vi "Image Manager for Grab Acquisition.vi"(7 "Mode":T4, 8 "error in (no error)":errorcluster, 9 "Init Settings":T3={"Number of Processing Images"=1, "Image Border Size"=0} {"Number of Processing Images" min=1 max=1000}, 10 "Image Settings In":cluster{"Image":T1, "Buffer Number":u32}, 11 "Session In":T2) -> (0 "error out":errorcluster, 1 "No Available Image":bool, 2 "Image Settings Out":cluster{"Image":T1, "Buffer Number":u32}, 3 "Session Out":T2)   [LabVIEW 2018]
uses:
  <vilib>/vision/Image Controls.llb/IMAQ Image.ctl
  Grab Manager Mode.ctl
  <vilib>/userDefined/High Color/IMAQdx.ctl
panel:
  in  "Invalid Image":errorcluster={"status"=TRUE, "code"=-2, "source"="The image passed in is not valid to Unlockl"}
  in  "Invalid Session":errorcluster={"status"=TRUE, "code"=-1, "source"="The images for this session are not available anymore."}
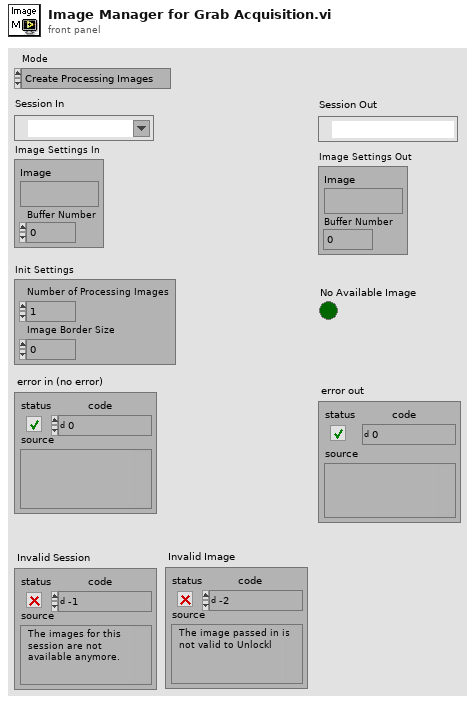
[diagram p1: front panel]
types:
  T1 = typedef "IMAQ Image.ctl" = refnum<image>
  T2 = typedef "IMAQdx.ctl" = refnum<k21>
  T3 = cluster{"Number of Processing Images":u32, "Image Border Size":u32}
  T4 = typedef "Grab Manager Mode.ctl" = enum16{"Create Processing Images", "Lock", "Add Acquired Image", "Get Acquired Image", "Unlock", "Dispose Processing Images"}
  T5 = cluster{cluster{"Image":T1, "Buffer Number":u32}[]}
  T6 = cluster{cluster{"Image":T1, "Buffer Number":u32}[]}[]
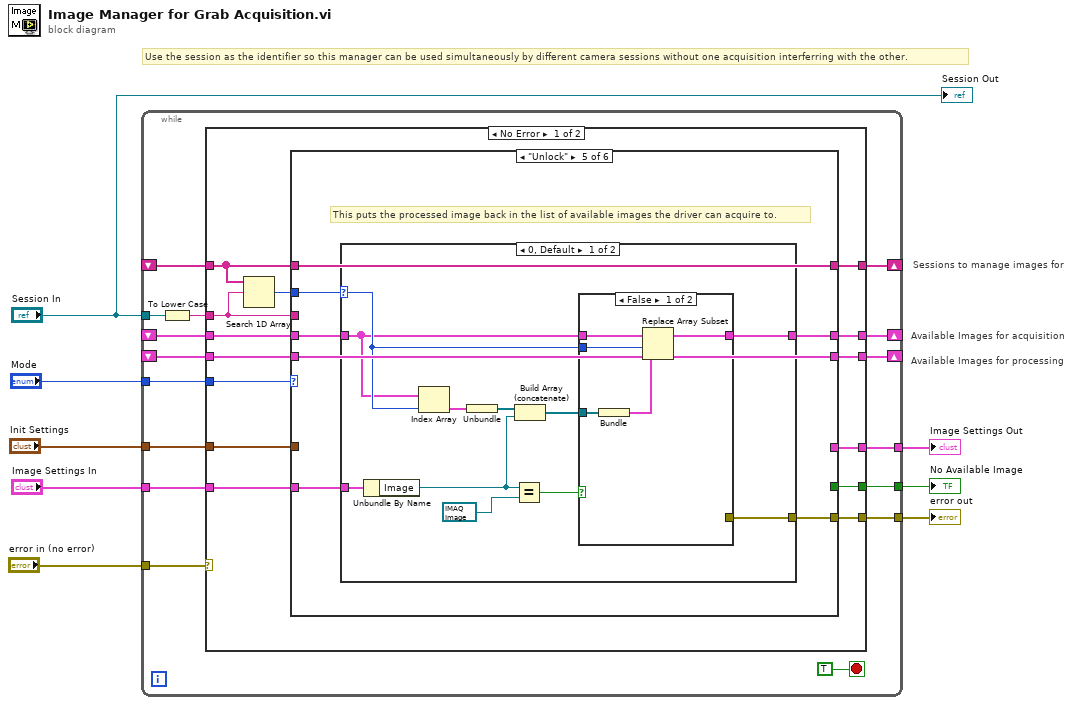
[diagram p0: block diagram]
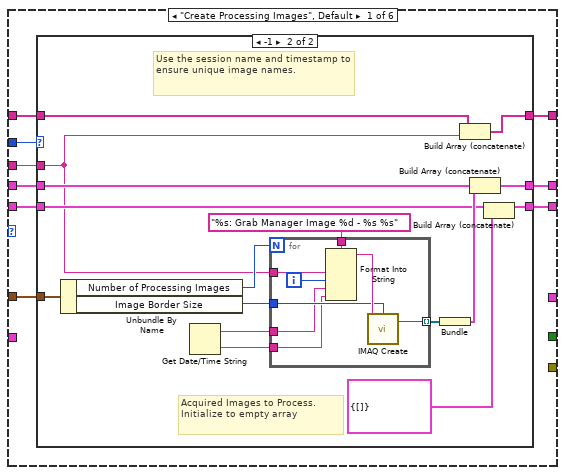
[diagram p2: hidden frame]
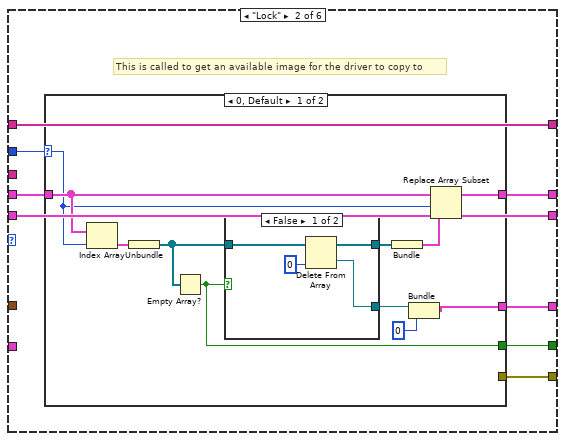
[diagram p4: hidden frame]
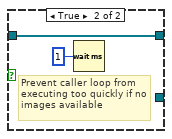
[diagram p5: hidden frame]
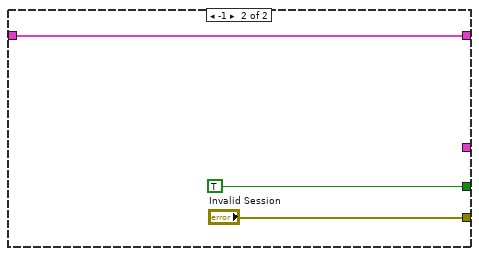
[diagram p6: hidden frame]
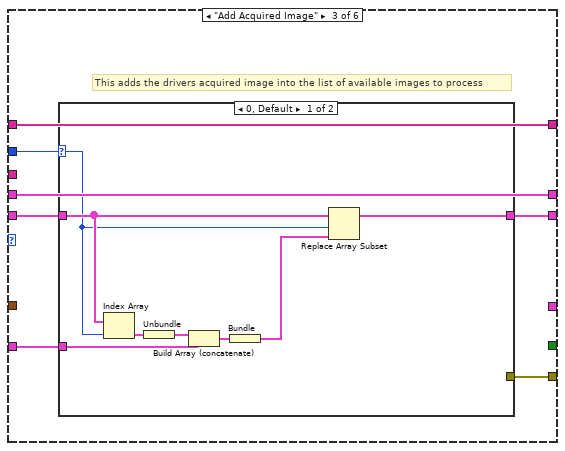
[diagram p7: hidden frame]
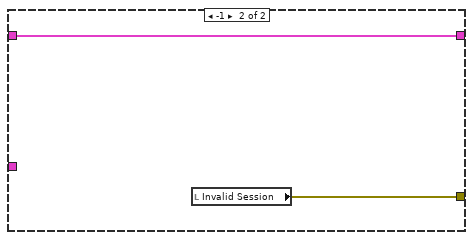
[diagram p8: hidden frame]
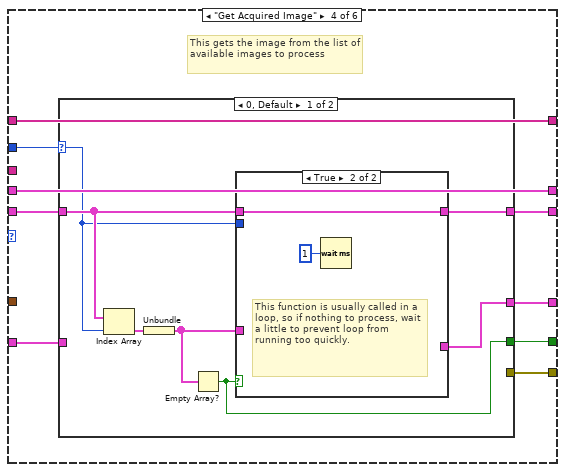
[diagram p9: hidden frame]
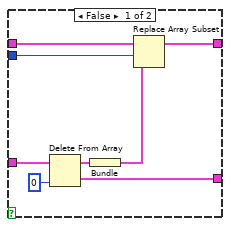
[diagram p10: hidden frame]
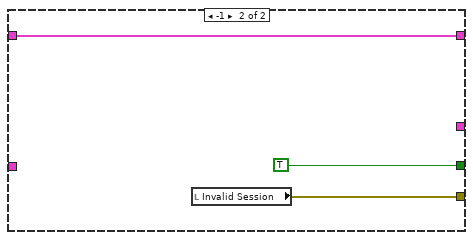
[diagram p11: hidden frame]
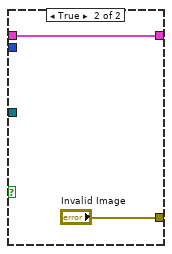
[diagram p12: hidden frame]
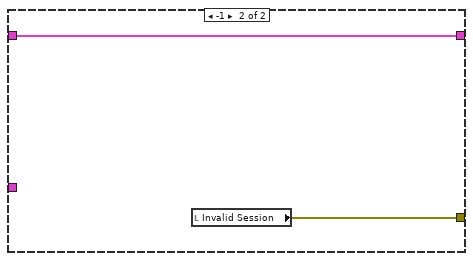
[diagram p13: hidden frame]
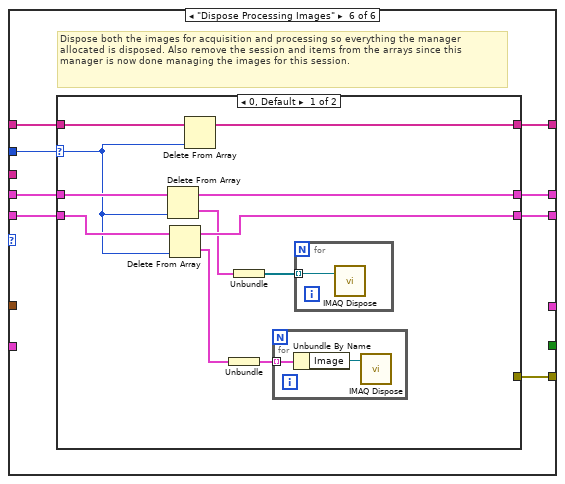
[diagram p14: hidden frame]
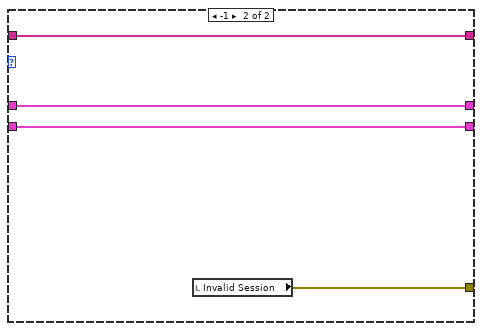
[diagram p15: hidden frame]
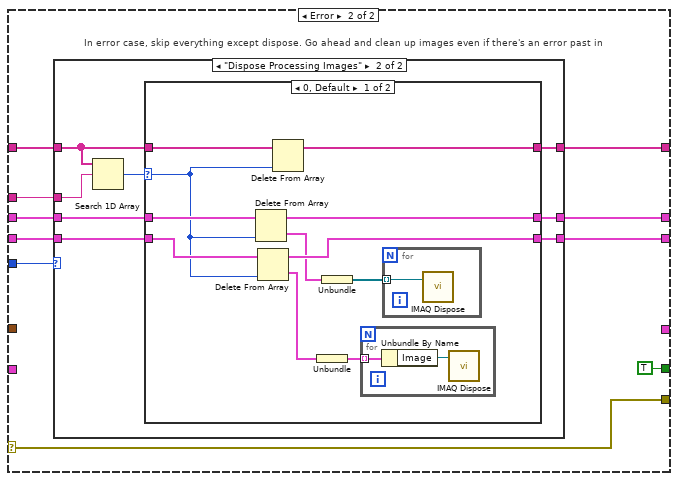
[diagram p16: hidden frame]
diagram:
  # "Use the session as the identifier so this manager can be used simultaneously by different camera sessions without one acquisition interferring with the other."
  # "Available Images for processing"
  # "Available Images for acquisition"
  # "Sessions to manage images for"
  n1 = while {
    tunnel: "Mode" -> [w24]
    tunnel: [w23] -> w7
    tunnel: "Session In" -> [w22]
    tunnel: "error in (no error)" -> [w20]
    tunnel: "Init Settings" -> [w19]
    shift-right: [w18] -> _
    shift-left: _ -> [w17]
    shift-right: [w16] -> _
    shift-left: _ -> [w15]
    tunnel: [w14] -> w3
    shift-right: [w13] -> _
    shift-left: _ -> [w12]
    tunnel: [w11] -> w1
    tunnel: "Image Settings In" -> [w10]
    stop <- TRUE stop-if-true
    n2 = To Lower Case(string=w22) -> (all lower case string=w9:string)
    n3 = case shown="No Error" w20 {
      selector: w20 -> [_ w211]
      tunnel: w24 -> [w38 w203]
      tunnel: [w37 _] -> w11
      tunnel: [w28 w211] -> w14
      tunnel: [w36 TRUE ("empty?")] -> w23
      tunnel: w9 -> [w34 w209]
      tunnel: w19 -> [w35 _]
      tunnel: [w33 w206] -> w18
      tunnel: w17 -> [w32 w210]
      tunnel: [w30 w205] -> w16
      tunnel: w15 -> [w29 w208]
      tunnel: [w27 w204] -> w13
      tunnel: w12 -> [w26 w207]
      tunnel: w10 -> [w25 _]
      frame No Error {
        n4 = Search 1D Array(1D array=w32, element=w34) -> (index of element=w31:i32)  [unwired: 1 in]
        n5 = case shown="\"Unlock\"" w38 {
          tunnel: [_ w75 _ w121 _ _] -> w37
          tunnel: [_ w82 _ w120 _ _] -> w36
          tunnel: w34 -> [w46 _ _ _ _ _]
          tunnel: w35 -> [w47 _ _ _ _ _]
          tunnel: [w45 w80 w108 w127 w154 w179] -> w33
          tunnel: w32 -> [w44 w80 w108 w127 w154 w180]
          tunnel: w31 -> [w43 w81 w109 w128 w155 w183]
          tunnel: [w42 w78 w107 w126 w150 w178] -> w30
          tunnel: w29 -> [w41 w79 w107 w126 w151 w182]
          tunnel: [_ w77 w104 w123 w153 w176] -> w28
          tunnel: [w40 w76 w105 w124 w149 w177] -> w27
          tunnel: w26 -> [w39 w76 w106 w125 w149 w181]
          tunnel: w25 -> [_ _ w103 w122 w152 _]
          frame "Create Processing Images", Default {
            n6 = case shown="-1" w43 {
              tunnel: w47 -> [_ w66]
              tunnel: w46 -> [_ w53]
              tunnel: [w50 w65] -> w45
              tunnel: w44 -> [w50 w64]
              tunnel: [w49 w59] -> w42
              tunnel: w41 -> [w49 w58]
              tunnel: [w48 w56] -> w40
              tunnel: w39 -> [w48 w55]
              frame 0, Default {
                # "This session has already been initialized. Keep the same images"
              }
              frame -1 {
                # "Acquired Images to Process. Initialize to empty array"
                # "Use the session name and timestamp to ensure unique image names."
                n7 = Unbundle By Name(w66) -> ("Number of Processing Images"=w63:u32, "Image Border Size"=w62:u32)
                n8 = Get Date/Time String() -> (date string=w52:string, time string=w51:string)  [unwired: 3 in]
                n9 = for {
                  N: w63 -> [_]
                  tunnel: [w74] -> w61 mode=indexing
                  tunnel: w53 -> [w71]
                  tunnel: w62 -> [w70]
                  tunnel: "%s: Grab Manager Image %d - %s %s" ("Image Name") -> [w69]
                  tunnel: w52 -> [w68]
                  tunnel: w51 -> [w67]
                  i -> [w73]
                  n10 = Format Into String(format string=w69, w71, w73, w68, w67) -> (resulting string=w72:string)  [unwired: 2 in, 1 out]
                  n11 = call "IMAQ Create"("Border Size"=w70, "Image Name"=w72) -> ("New Image"=w74:T1)  [unwired: 2 in, 2 out]
                }
                n12 = Bundle(w61) -> (w60:cluster{T1[]})  [unwired: 1 in]
                n13 = Build Array (concatenate)(w64, w53) -> (w65:string[])
                n14 = Build Array (concatenate)(w58, w60) -> (w59:cluster{T1[]}[])
                n15 = Build Array (concatenate)(w55, T5 {[]}) -> (w56:T6)
              }
            }
          }
          frame "Lock" {
            # "This is called to get an available image for the driver to copy to"
            n16 = case shown="0, Default" w81 {
              selector: w81 -> [w87 _]
              tunnel: [w93 TRUE ("empty?")] -> w82
              tunnel: w79 -> [w89 w102]
              tunnel: [w88 w102] -> w78
              tunnel: [_ "Invalid Session"] -> w77
              tunnel: [w83 _] -> w75
              frame 0, Default {
                n17 = Index Array(array=w89, index=w87) -> (element=w92:cluster{T1[]})
                n18 = Unbundle(w92) -> (w91:T1[])
                n19 = Empty Array?(array=w91) -> (empty?=w93:bool)
                n20 = case shown="False" w93 {
                  tunnel: [w96 w99] -> w90
                  tunnel: [w95 _] -> w85
                  tunnel: w91 -> [w94 w99]
                  frame False {
                    n21 = Delete From Array(array=w94, index=0) -> (deleted portion=w95:T1, array with subset deleted=w96:T1[])  [unwired: 1 in]
                  }
                  frame True {
                    # "Prevent caller loop from executing too quickly if no images available"
                    n22 = Wait (ms)(milliseconds to wait=u32 1) -> ()  [unwired: 1 out]
                  }
                }
                n23 = Bundle(w90) -> (w86:cluster{T1[]})  [unwired: 1 in]
                n24 = Bundle("New Image"=w85, u32 0) -> (w83:cluster{"New Image":T1, u32})  [unwired: 1 in]
                n25 = Replace Array Subset(array=w89, new element=w86, index=w87) -> (w88:cluster{T1[]}[])
              }
              frame -1 {
              }
            }
          }
          frame "Add Acquired Image" {
            # "This adds the drivers acquired image into the list of available images to process"
            n26 = case shown="0, Default" w109 {
              selector: w109 -> [w112 _]
              tunnel: w106 -> [w115 w119]
              tunnel: [w111 w119] -> w105
              tunnel: [_ w118] -> w104
              tunnel: w103 -> [w110 _]
              frame 0, Default {
                n27 = Index Array(array=w115, index=w112) -> (element=w117:T5)
                n28 = Unbundle(w117) -> (w116:cluster{"Image":T1, "Buffer Number":u32}[])
                n29 = Build Array (concatenate)(w116, w110) -> (w114:cluster{"Image":T1, "Buffer Number":u32}[])
                n30 = Bundle(w114) -> (w113:T5)  [unwired: 1 in]
                n31 = Replace Array Subset(array=w115, new element=w113, index=w112) -> (w111:T6)
              }
              frame -1 {
                n32 = local read "Invalid Session"() -> (w118:errorcluster)
              }
            }
          }
          frame "Get Acquired Image" {
            # "This gets the image from the list of available images to process"
            n33 = case shown="0, Default" w128 {
              selector: w128 -> [w133 _]
              tunnel: w125 -> [w134 w148]
              tunnel: [w132 w148] -> w124
              tunnel: [_ w147] -> w123
              tunnel: w122 -> [_ _]
              tunnel: [w130 _] -> w121
              tunnel: [w129 TRUE ("empty?")] -> w120
              frame 0, Default {
                n34 = Index Array(array=w134, index=w133) -> (element=w135:T5)
                n35 = Unbundle(w135) -> (w131:cluster{"Image":T1, "Buffer Number":u32}[])
                n36 = Empty Array?(array=w131) -> (empty?=w129:bool)
                n37 = case shown="True" w129 {
                  tunnel: w134 -> [w143 w145]
                  tunnel: w133 -> [w142 _]
                  tunnel: [w141 w145] -> w132
                  tunnel: w131 -> [w139 _]
                  tunnel: [w136 _] -> w130
                  frame False {
                    n38 = Delete From Array(array=w139, index=0) -> (deleted portion=w136:cluster{"Image":T1, "Buffer Number":u32}, array with subset deleted=w138:cluster{"Image":T1, "Buffer Number":u32}[])  [unwired: 1 in]
                    n39 = Bundle(w138) -> (w137:T5)  [unwired: 1 in]
                    n40 = Replace Array Subset(array=w143, new element=w137, index=w142) -> (w141:T6)
                  }
                  frame True {
                    # "This function is usually called in a loop, so if nothing to process, wait a little to prevent loop from running too quickly."
                    n41 = Wait (ms)(milliseconds to wait=u32 1) -> ()  [unwired: 1 out]
                  }
                }
              }
              frame -1 {
                n42 = local read "Invalid Session"() -> (w147:errorcluster)
              }
            }
          }
          frame "Unlock" {
            # "This puts the processed image back in the list of available images the driver can acquire to."
            n43 = case shown="0, Default" w155 {
              selector: w155 -> [w165 _]
              tunnel: [w156 w175] -> w153
              tunnel: w152 -> [w166 _]
              tunnel: w151 -> [w161 w174]
              tunnel: [w160 w174] -> w150
              frame 0, Default {
                n44 = Unbundle By Name(w166) -> ("Image"=w159:T1)
                n45 = Index Array(array=w161, index=w165) -> (element=w164:cluster{T1[]})
                n46 = Unbundle(w164) -> (w163:T1[])
                n47 = Equal?(x=w159, y=T1 refnum) -> (x = y?=w157:bool)
                n48 = Build Array (concatenate)(w163, w159) -> (w162:T1[])
                n49 = case shown="False" w157 {
                  tunnel: w165 -> [w171 _]
                  tunnel: w162 -> [w169 _]
                  tunnel: w161 -> [w168 w173]
                  tunnel: [w167 w173] -> w160
                  tunnel: [_ "Invalid Image"] -> w156
                  frame False {
                    n50 = Bundle(w169) -> (w170:cluster{T1[]})  [unwired: 1 in]
                    n51 = Replace Array Subset(array=w168, new element=w170, index=w171) -> (w167:cluster{T1[]}[])
                  }
                  frame True {
                  }
                }
              }
              frame -1 {
                n52 = local read "Invalid Session"() -> (w175:errorcluster)
              }
            }
          }
          frame "Dispose Processing Images" {
            # "Dispose both the images for acquisition and processing so everything the manager allocated is disposed. Also remove the session and items from the arrays since this manager is now done managing the images for this session."
            n53 = case shown="0, Default" w183 {
              selector: w183 -> [w188 _]
              tunnel: w182 -> [w191 w199]
              tunnel: w181 -> [w189 w198]
              tunnel: w180 -> [w193 w200]
              tunnel: [w192 w200] -> w179
              tunnel: [w190 w199] -> w178
              tunnel: [w187 w198] -> w177
              tunnel: [_ w201] -> w176
              frame 0, Default {
                n54 = Delete From Array(array=w191, index=w188) -> (deleted portion=w186:cluster{T1[]}, array with subset deleted=w190:cluster{T1[]}[])  [unwired: 1 in]
                n55 = Delete From Array(array=w189, index=w188) -> (deleted portion=w185:T5, array with subset deleted=w187:T6)  [unwired: 1 in]
                n56 = Delete From Array(array=w193, index=w188) -> (array with subset deleted=w192:string[])  [unwired: 1 in, 1 out]
                n57 = Unbundle(w185) -> (w184:cluster{"Image":T1, "Buffer Number":u32}[])
                n58 = Unbundle(w186) -> (w194:T1[])
                n59 = for {
                  tunnel: w184 -> [w196] mode=indexing
                  n60 = Unbundle By Name(w196) -> ("Image"=w195:T1)
                  n61 = call "IMAQ Dispose"("Image"=w195) -> ()  [unwired: 5 in, 1 out]
                }
                n62 = for {
                  tunnel: w194 -> [w197] mode=indexing
                  n63 = call "IMAQ Dispose"("Image"=w197) -> ()  [unwired: 5 in, 1 out]
                }
              }
              frame -1 {
                n64 = local read "Invalid Session"() -> (w201:errorcluster)
              }
            }
          }
        }
      }
      frame Error {
        # "In error case, skip everything except dispose. Go ahead and clean up images even if there's an error past in"
        n65 = case shown="\"Dispose Processing Images\"" w203 {
          tunnel: w210 -> [w214 w222]
          tunnel: w209 -> [_ w221]
          tunnel: w208 -> [w213 w219]
          tunnel: w207 -> [w212 w218]
          tunnel: [w214 w217] -> w206
          tunnel: [w213 w216] -> w205
          tunnel: [w212 w215] -> w204
          frame Default {
          }
          frame "Dispose Processing Images" {
            n66 = Search 1D Array(1D array=w222, element=w221) -> (index of element=w220:i32)  [unwired: 1 in]
            n67 = case shown="0, Default" w220 {
              selector: w220 -> [w227 _]
              tunnel: w219 -> [w230 w238]
              tunnel: w218 -> [w228 w237]
              tunnel: w222 -> [w232 w239]
              tunnel: [w231 w239] -> w217
              tunnel: [w229 w238] -> w216
              tunnel: [w226 w237] -> w215
              frame 0, Default {
                n68 = Delete From Array(array=w230, index=w227) -> (deleted portion=w225:cluster{T1[]}, array with subset deleted=w229:cluster{T1[]}[])  [unwired: 1 in]
                n69 = Delete From Array(array=w228, index=w227) -> (deleted portion=w224:T5, array with subset deleted=w226:T6)  [unwired: 1 in]
                n70 = Delete From Array(array=w232, index=w227) -> (array with subset deleted=w231:string[])  [unwired: 1 in, 1 out]
                n71 = Unbundle(w224) -> (w223:cluster{"Image":T1, "Buffer Number":u32}[])
                n72 = Unbundle(w225) -> (w233:T1[])
                n73 = for {
                  tunnel: w223 -> [w235] mode=indexing
                  n74 = Unbundle By Name(w235) -> ("Image"=w234:T1)
                  n75 = call "IMAQ Dispose"("Image"=w234) -> ()  [unwired: 5 in, 1 out]
                }
                n76 = for {
                  tunnel: w233 -> [w236] mode=indexing
                  n77 = call "IMAQ Dispose"("Image"=w236) -> ()  [unwired: 5 in, 1 out]
                }
              }
              frame -1 {
              }
            }
          }
        }
      }
    }
  }
  "error out" <- w3
  "No Available Image" <- w7
  "Image Settings Out" <- w1
  "Session Out" <- "Session In"
